vi "STA - Wave V5 Host_ohnedt.vi"() -> ()   [LabVIEW 2015]
doc: "The continuous acquisition mode tells the FPGA to acquire points indefinitely until a stop command is issued or until an error is encountered (FIFO overflow, module underflow, and so on). \n\nIn this acquisition mode, explicitly call the appropriate rwfm_ConfigTiming VI and set the host application's data buffer to be many times larger than the read size. The examples use a 10X size by default. If the host application's data buffer fills, then the FPGA experiences a FIFO overflow causing the acquisition to stop."
uses:
  <vilib>/LabVIEW Targets/FPGA/cRIO/shared/nicrio_ModuleControls/nicrio_cRIO-9234_ConfigModeRing.ctl
  <vilib>/FPGAPlugInAG/cRIO-9112/niLvFpga_Open_cRIO-9112.vi
  <vilib>/rvi/interface/common/dynamic/niFpgaDynamicAddResources.vi
  <vilib>/Utility/error.llb/Error Cluster From Error Code.vi
  <vilib>/RVI Host/nirviSupport.llb/nirviErrorClusterFromErrorCode.vi
  <vilib>/rvi/errors/niLvFpgaAdjustHostInterfaceError.vi
  <vilib>/FPGAPlugInAG/Dynamic/niLvFpga_Close_Dynamic.vi
  <vilib>/rvi/interface/nirviOpenFPGA/nirviOpenFPGA.xnode
  STA - Waveform V5/FPGA Bitfiles/STA-WaveformV5_FPGATarget2_[FPGA]DeltaSigMa_1aVPXft62yI.lvbitx
  STA - Waveform V5/FPGA/[FPGA] DeltaSig Main V5.vi
  <vilib>/rvi/interface/nirviMethod/nirviMethod.xnode
  <vilib>/rvi/interface/nirviCloseFPGA/nirviCloseFPGA.xnode
  <vilib>/NI/cRIO Wfm/cRIO Wfm.lvlib
  D/Documents/LabVIEW Data/STA - Waveform V0/FPGA Bitfiles/SARAcqMain_9074.lvbitx
  C:/Program Files (x86)/National Instruments/LabVIEW 2015/ProjectTemplates/Source/cRIOWfm/FPGA/[FPGA] SAR Acq Main.vi
  <vilib>/rvi/interface/nirviMethod/StockFPGA_InlinedMethodWaitForSingleIRQ.vi
  <vilib>/FPGAPlugInAG/Dynamic/niLvFpga_WaitOnIrq_Dynamic.vi
panel:
  out "Time Measure":dbl
  out "data rate (S/s)":u32
  out "Channel Config":T2(array[cluster]) {"Input Configuration" items=["AC Coupled", "DC Coupled", "IEPE AC Coupled"]}
  out "Samples per Read":i32
  out "file path":path
  in  "error in (no error)":errorcluster
  out "error out":errorcluster
  in  "stop":bool
  out "Waveform Graph":waveform(sgl)[](graph)
  out "Buffer Backlog":dbl caption="RT Buffer Backlog [%]" format="%#.2g"
  # "Sampling Info"
  # "Channel Info"
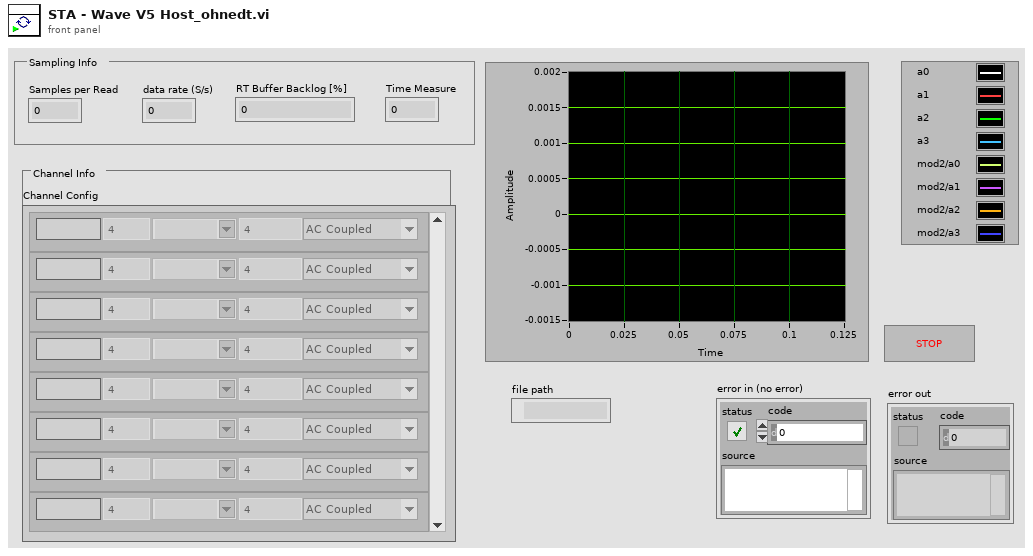
[diagram p1: front panel]
types:
  T1 = typedef "nicrio_cRIO-9234_ConfigModeRing.ctl" = u8
  T2 = cluster{"Channel Name":string, "Sensitivity mV_EU":dbl, "EU":string, "Input Configuration":T1, "dB Ref EU":dbl}[]
  T3 = enum16{"open", "open or create", "create or replace", "create", "open (read-only)"}
  T4 = typedef "Acquisition and Logging Configuration_Waveform.ctl" = cluster{"Data Rate":T5, "Samples per Read":i32, "Number of Reads to Save":i32, "Data File Name":string, "TDMS Properties":T6[], "Number of Channels":i32, "Trigger - RMS Value":dbl, "Trigger - Channel":i32, "Trigger - Time (Minute)":i32, "Channel Config":cluster{"Channel Name":string, "Sensitivity mV_EU":dbl, "EU":string, "Input Configuration":T1, "dB Ref EU":dbl}[], "data rate (S/s)":u32, "Time Measure":dbl}
  T5 = typedef "nicrio_cRIO-9234_DataRatesRing2.ctl" = u8
  T6 = typedef "TDMS Properties.ctl" = cluster{"Name":string, "Value":string}
  T7 = typedef "cRIO Wfm.lvlib/SamplingInfo.ctl" = cluster{"Number of Channels":i32, "Actual Samp Rate":dbl, "Chan Name Array":string[], "EU Chan Array":string[], "dB Ref Chan Array":dbl[]}
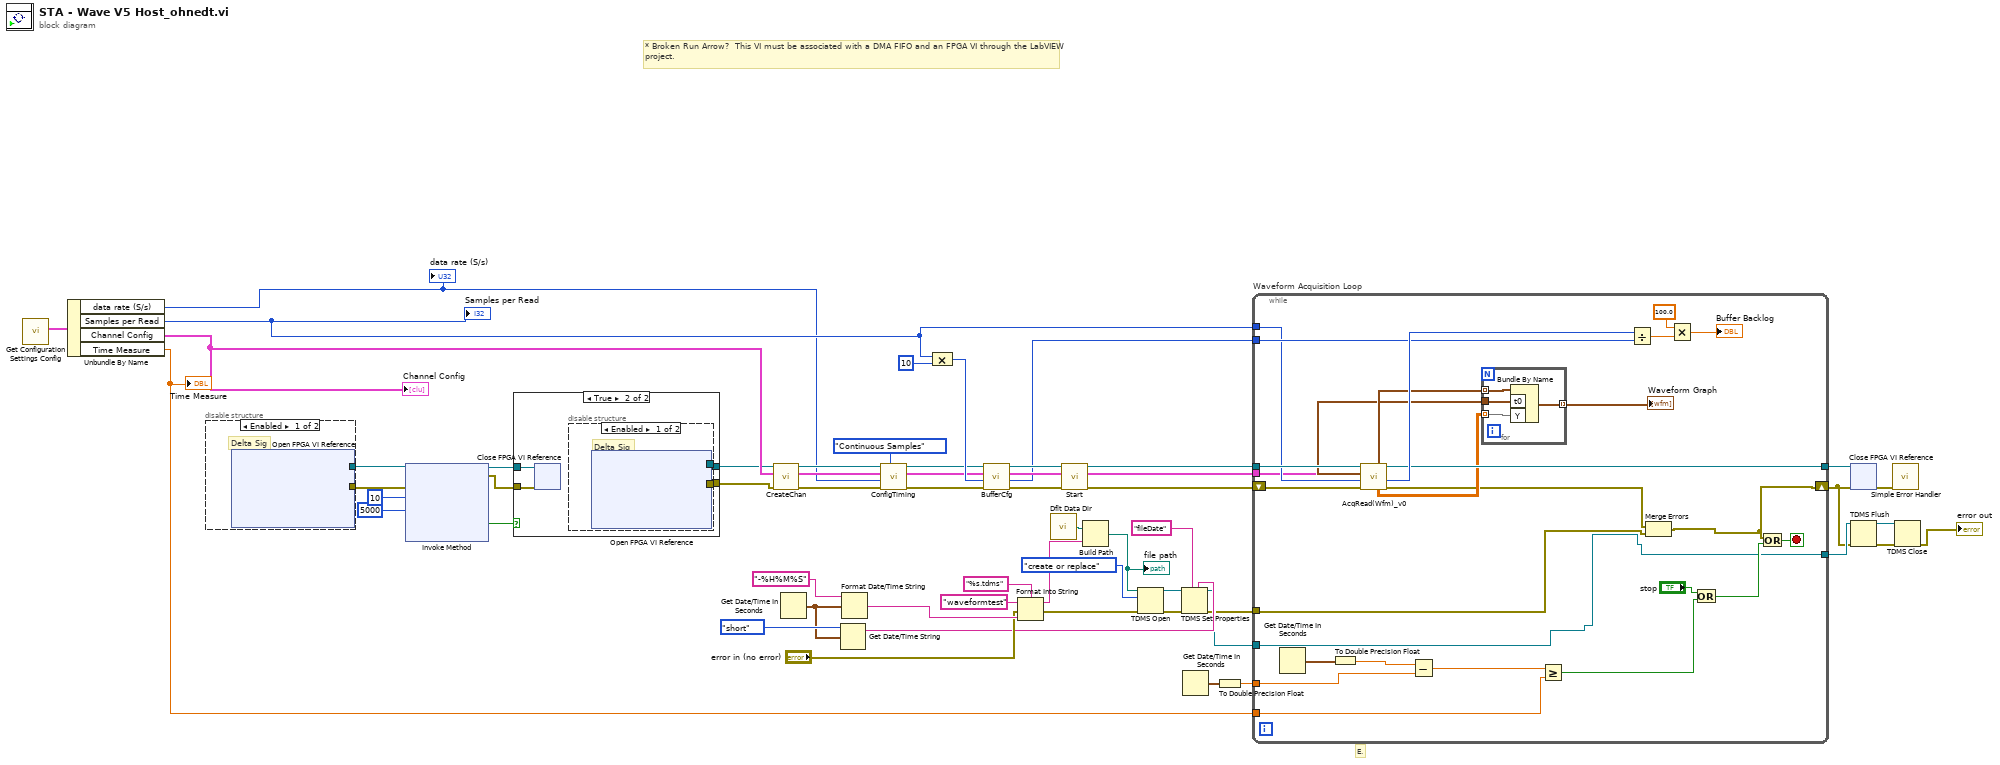
[diagram p0: block diagram]
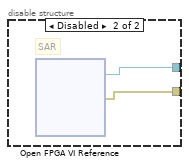
[diagram p3: hidden frame]
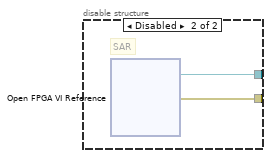
[diagram p4: hidden frame]
diagram:
  # "E."
  # "* Broken Run Arrow?  This VI must be associated with a DMA FIFO and an FPGA VI through the LabVIEW project."
  n1 = call "Get Configuration Settings Config.vi"() -> ("Configuration"=w17:T4)  [unwired: 10 in, 1 out]
  n2 = Unbundle By Name(w17) -> ("data rate (S/s)"=w14:u32, "Samples per Read"=w16:i32, "Channel Config"=w15:T2, "Time Measure"=w2:dbl)
  "Samples per Read" <- w16
  "Channel Config" <- w15
  "data rate (S/s)" <- w14
  "Time Measure" <- w2
  n3 = disable-structure shown="Enabled" {
    disable-tunnel: [w59 w61] -> w11
    disable-tunnel: [w58 w60] -> w10
    frame Enabled {
      # "Delta Sig"
      n4 = xnode "Open FPGA VI Reference"() -> ("FPGA VI Reference Out"=w59:refnum<k20>, "error out"=w58:errorcluster)  [unwired: 2 in]
    }
    frame Disabled {
      # "SAR"
      n5 = xnode "Open FPGA VI Reference"() -> ("FPGA VI Reference Out"=w61:refnum<k20>, "error out"=w60:errorcluster)  [unwired: 2 in]
    }
  }
  n6 = xnode "Invoke Method"("FPGA VI Reference In"=w11, "error in"=w10, "IRQ Number(s)"=10, "Timeout (ms)"=5000) -> ("FPGA VI Reference Out"=w8:refnum<k20>, "error out"=w7:errorcluster, "Timed Out"=w9:bool)  [unwired: 1 out]
  n7 = case shown="True" w9 {
    tunnel: w8 -> [w63 w67]
    tunnel: w7 -> [w62 w66]
    tunnel: [w63 w65] -> w1
    tunnel: [w62 w64] -> w6
    frame False {
    }
    frame True {
      n8 = xnode "Close FPGA VI Reference"("FPGA VI Reference In"=w67, "error in"=w66) -> ()  [unwired: 1 out]
      n9 = disable-structure shown="Enabled" {
        disable-tunnel: [w69 w71] -> w65
        disable-tunnel: [w68 w70] -> w64
        frame Enabled {
          # "Delta Sig"
          n10 = xnode "Open FPGA VI Reference"() -> ("FPGA VI Reference Out"=w69:refnum<k20>, "error out"=w68:errorcluster)  [unwired: 2 in]
        }
        frame Disabled {
          # "SAR"
          n11 = xnode "Open FPGA VI Reference"() -> ("FPGA VI Reference Out"=w71:refnum<k20>, "error out"=w70:errorcluster)  [unwired: 2 in]
        }
      }
    }
  }
  n12 = call <vilib>:"CreateChan.vi"("Dynamic FPGA Ref"=w1, "Channel Config"=w15, "error in"=w6) -> ("Dynamic FPGA Ref Out"=w46:refnum<k20>, "Sampling Info"=w45:T7, "error out"=w41:errorcluster)  [unwired: 5 in]
  n13 = Get Date/Time In Seconds() -> (seconds since 1Jan1904=w5:timestamp)
  n14 = Get Date/Time String(date format (0)=enum16{"short", "long", "abbreviated"}."short", seconds (now)=w5) -> (date string=w25:string)  [unwired: 1 in, 1 out]
  n15 = Format Date/Time String(time format string (%c)="-%H%M%S", seconds (now)=w5) -> (date/time string=w35:string)  [unwired: 1 in]
  n16 = call <vilib>:"ConfigTiming.vi"("Sample Mode"=enum16{"Finite Samples", "Continuous Samples"}."Continuous Samples", "error in"=w41, "Sample Rate"=w14, "Sampling Info In"=w45, "Dynamic FPGA Ref"=w46) -> ("error out"=w42:errorcluster, "Sampling Info Out"=w43:T7, "Dynamic FPGA Ref Out"=w44:refnum<k20>)  [unwired: 3 in, 1 out]
  n17 = Compound Arithmetic op=MULTIPLY(w16, 10 ("value")) -> (w50:i32)
  n18 = call <vilib>:"BufferCfg.vi"("error in"=w42, "Buffer Size [Samps per Chan]"=w50, "Sampling Info In"=w43, "Dynamic FPGA Ref"=w44) -> ("error out"=w51:errorcluster, "Buffer Size [Total Samples]"=w47:u32, "Sampling Info Out"=w49:T7, "Dynamic FPGA Ref Out"=w52:refnum<k20>)  [unwired: 4 out]
  n19 = Format Into String(format string="%s.tdms", initial string="waveformtest", error in="error in (no error)", w35) -> (resulting string=w39:string, error out=w23:errorcluster)
  n20 = call <vilib>:"Dflt Data Dir.vi"() -> ("App:Default Data Directory"=w32:path)
  n21 = call <vilib>:"Start.vi"("error in"=w51, "Sampling Info In"=w49, "Dynamic FPGA Ref"=w52) -> ("error out"=w56:errorcluster, "Sampling Info Out"=w48:T7, "Dynamic FPGA Ref Out"=w57:refnum<k20>)  [unwired: 6 out]
  n22 = Build Path(base path=w32, name or relative path=w39) -> (appended path=w28:path)
  "file path" <- w28
  n23 = TDMS Open(8:w23, 10:T3."create or replace" ("operation (0:open)"), 11:w28) -> (0:w31:errorcluster, 3:w30:refnum<k34>)  [unwired: 4 in]
  n24 = TDMS Set Properties(5:w25, 7:"fileDate" ("property names"), 8:w31, 11:w30) -> (0:w21:errorcluster, 3:w22:refnum<k34>)  [unwired: 2 in, 2 out]
  n25 = Get Date/Time In Seconds() -> (seconds since 1Jan1904=w3:timestamp)
  n26 = To Double Precision Float(number=w3) -> (double precision float=w4:dbl)
  n27 = while "Waveform Acquisition Loop" {
    tunnel: w57 -> [w92]
    tunnel: [w89] -> w55
    tunnel: w48 -> [w85]
    tunnel: w47 -> [w96]
    tunnel: w16 -> [w90]
    shift-right: [w83] -> w19
    shift-left: w56 -> [w98]
    tunnel: w22 -> [w73]
    tunnel: w21 -> [w72]
    tunnel: [w73] -> w20
    tunnel: w4 -> [w75]
    tunnel: w2 -> [w74]
    stop <- w91 stop-if-true
    n28 = Get Date/Time In Seconds() -> (seconds since 1Jan1904=w77:timestamp)
    n29 = To Double Precision Float(number=w77) -> (double precision float=w76:dbl)
    n30 = call <vilib>:"AcqRead(Wfm)_v0.vi"("error in"=w98, "Samps Read per Chan"=w90, "Sampling Info"=w85, "Dynamic FPGA Ref"=w92) -> ("error out"=w84:errorcluster, "Samples Remaining"=w97:u32, "time stamp"=w86:timestamp, "Dynamic FPGA Ref Out"=w89:refnum<k20>, "transposed array"=w87:sgl[][], "Array"=w88:waveform(sgl)[])  [unwired: 2 in]
    n31 = Subtract(x=w76, y=w75) -> (x-y=w78:dbl)
    n32 = for {
      tunnel: w88 -> [w102] mode=indexing
      tunnel: w86 -> [w101]
      tunnel: [w100] -> w82 mode=indexing
      tunnel: w87 -> [w99] mode=indexing
      n33 = Bundle By Name(cluster=w102, "t0"=w101, "Y"=w99) -> (w100:waveform(sgl))
    }
    "Waveform Graph" <- w82
    n34 = Greater Or Equal?(x=w78, y=w74) -> (x >= y?=w81:bool)
    n35 = Divide(x=w97, y=w96) -> (x/y=w95:dbl)
    n36 = Merge Errors(w84, w72) -> (w83:errorcluster)
    n37 = Multiply(x=100.0, y=w95) -> (x*y=→"Buffer Backlog":dbl)
    n38 = Or(x="stop", y=w81) -> (x .or. y?=w79:bool)
    n39 = Or(x=w83, y=w79) -> (x .or. y?=w91:bool)
  }
  n40 = xnode "Close FPGA VI Reference"("FPGA VI Reference In"=w55, "error in"=w19) -> ("error out"=w53:errorcluster)
  n41 = TDMS Flush(4:w19, 7:w20) -> (0:w29:errorcluster, 3:w18:refnum<k34>)
  n42 = call <vilib>:"Simple Error Handler.vi"("error in (no error)"=w53) -> ()  [unwired: 1 in, 8 out]
  n43 = TDMS Close(8:w29, 11:w18) -> (0:→"error out":errorcluster)  [unwired: 1 out]
